vi "teleop.vi"() -> ()   [LabVIEW 2010]
uses:
  <vilib>/NXT/Dual Mode Library/Display/drawNumber.vi
  <vilib>/NXT/Dual Mode Library/Waits/Wait_Num.vi
  Remote Interface/Remote Interface.lvlib
panel:
  in  "Total Loops (lagometer)":i32
  out "Enabled?":enum16{"Disabled", "Enabled"}(ring)
types:
  T1 = typedef "LVHSConnector.ctl" = cluster{"Hardware":string, "Flattened String":string}
  T2 = cluster{"4134 Button ID":enum16{"1-1", "1-2", "1-3", "1-4", "1-5", "1-6", "1-7", "1-8", "1-9", "1-10", "1-11", "1-12", "2-1", "2-2", "2-3", "2-4", "2-5", "2-6", "2-7", "2-8", "2-9", "2-10", "2-11", "2-12", "NXT-L", "NXT-R", "NXT-E", "1-U", "1-UR", "1-R", "1-DR", "1-D", "1-DL", "1-L", "1-UL", "2-U", "2-UR", "2-R", "2-DR", "2-D", "2-DL", "2-L", "2-UL"}, "4134 Event Type":enum16{"Pressed", "Released", "Toggled", "Untoggled"}}[]
  T3 = enum16{"Pressed", "Released", "Toggled", "Untoggled"}
  T4 = enum16{"None", "Left Button", "Right Button", "Enter Button"}
  T5 = enum16{"None", "Button 1", "Button 2", "Button 3", "Button 4", "Button 5", "Button 6", "Button 7", "Button 8", "Button 9", "Button 10", "Button 11", "Button 12", "POV Up", "POV Up Right", "POV Right", "POV Down Right", "POV Down", "POV Down Left", "POV Left", "POV Up Left"}
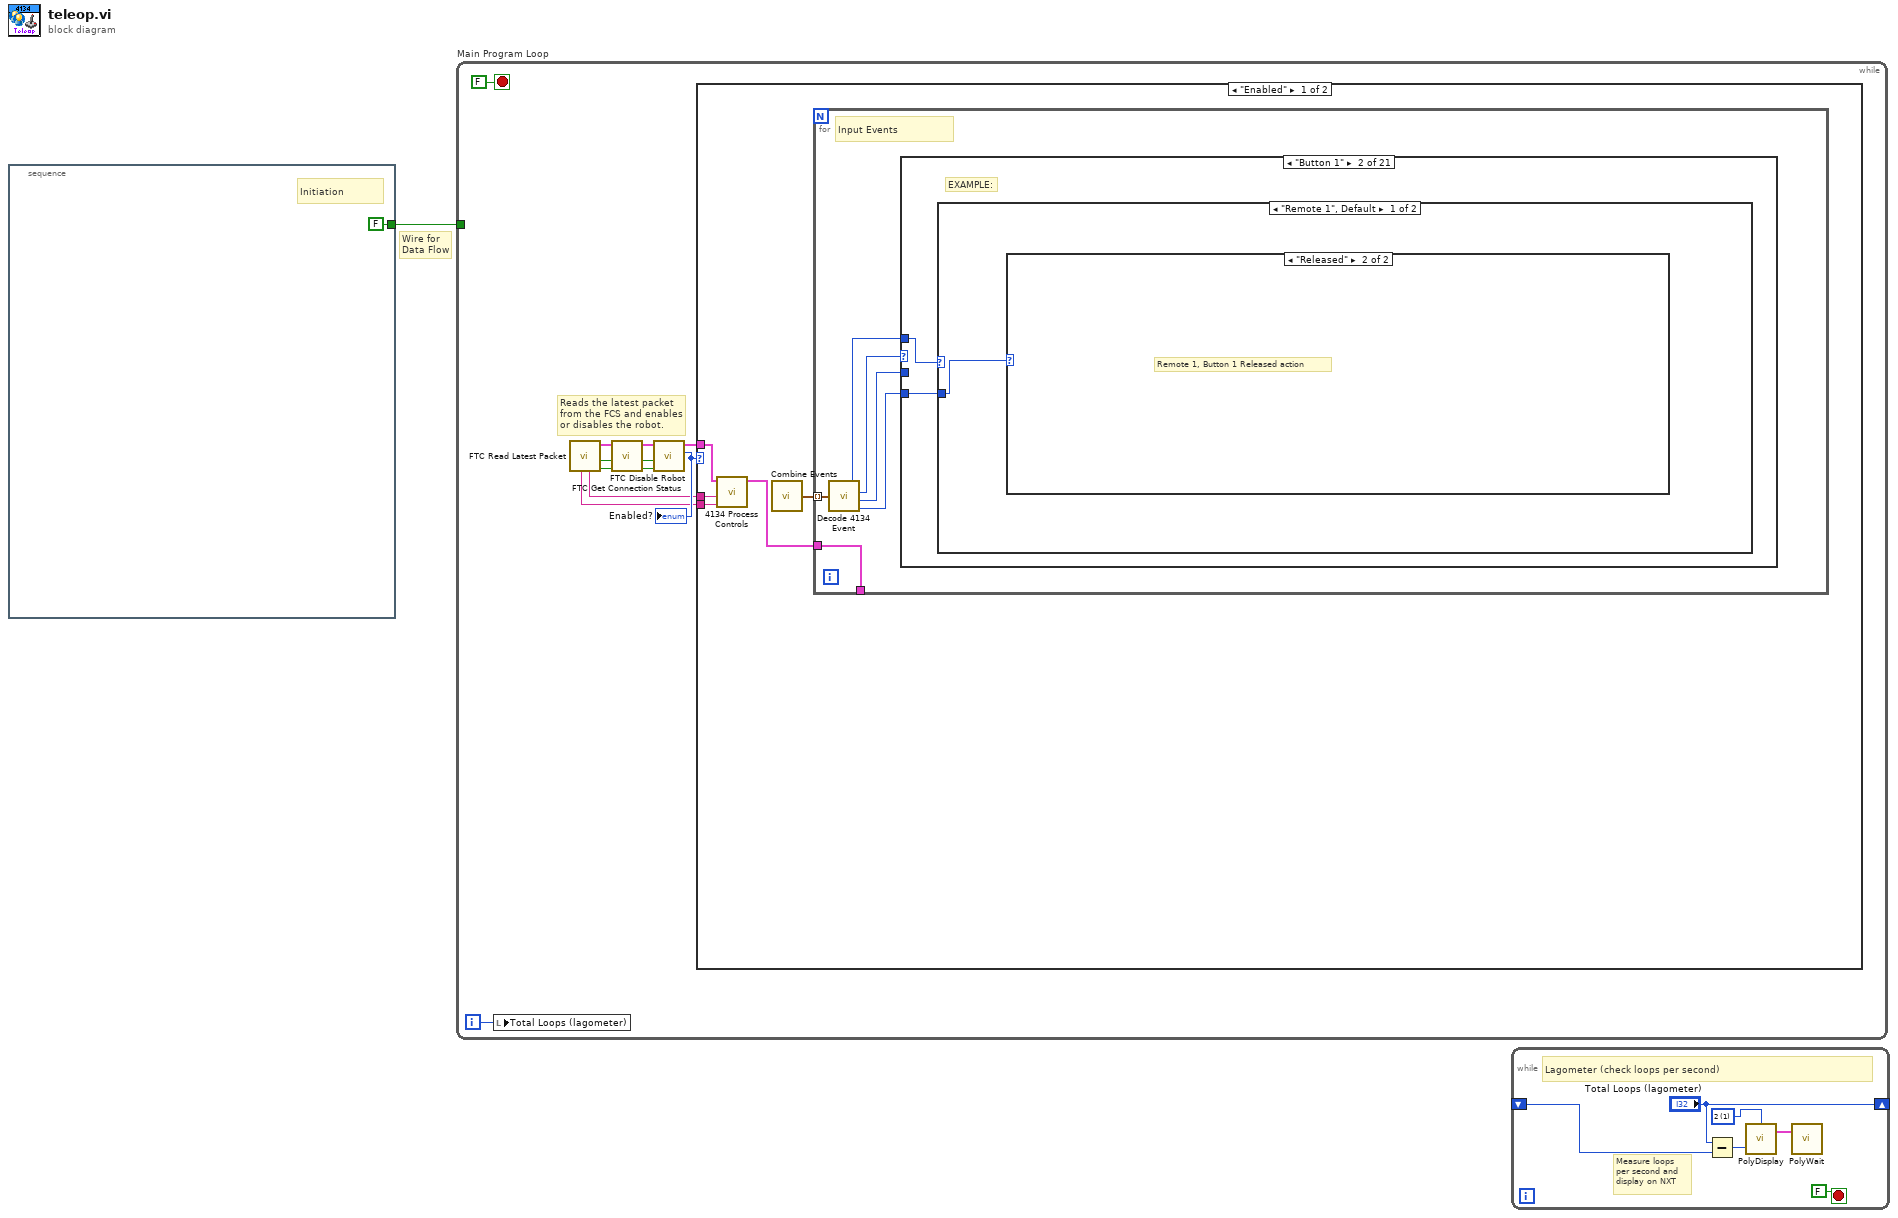
[diagram p0: block diagram]
diagram:
  # "Wire for\nData Flow"
  n1 = stacked-sequence {
    tunnel: [FALSE] -> w1
    frame #0 {
      # "Initiation"
    }
  }
  n2 = while "Main Program Loop" {
    tunnel: w1 -> [_]
    i -> [w3]
    stop <- FALSE stop-if-true
    # "Reads the latest packet\nfrom the FCS and enables\nor disables the robot."
    n3 = local write "Total Loops (lagometer)"(w3) -> ()
    n4 = call <vilib>:"FTC Read Latest Packet.vi"() -> ("Packet Received?"=w13:bool, "Stopped?"=w10:bool, "NXT"=w12:T1, "Controller 1"=w5:string, "Controller 2"=w4:string)  [unwired: 6 in, 1 out]
    n5 = call <vilib>:"FTC Get Connection Status.vi"("Packet Received?"=w13, "Stopped?"=w10, "NXT"=w12) -> ("Online?"=w7:bool, "Stopped?"=w8:bool, "NXT"=w9:T1)  [unwired: 5 in]
    n6 = call <vilib>:"FTC Disable Robot.vi"("Online?"=w7, "Stopped?"=w8, "NXT"=w9) -> ("Enabled?"=w11:enum16{"Disabled", "Enabled"}, "NXT"=w6:T1)  [unwired: 3 in]
    "Enabled?" <- w11
    n7 = case "disableCase" shown="\"Enabled\"" w11 {
      tunnel: w5 -> [w19 _]
      tunnel: w4 -> [w18 _]
      tunnel: w6 -> [w17 w34]
      frame "Enabled" {
        n8 = call "4134 Process Controls.vi"("Remote 2 Packet"=w18, "Remote 1 Packet"=w19, "NXT"=w17) -> ("NXT"=w15:T1)  [unwired: 6 in, 2 out]
        n9 = call "Combine Events.vi"() -> ("4134 Events"=w16:T2)  [unwired: 2 in]
        n10 = for {
          tunnel: w16 -> [w25] mode=indexing
          tunnel: w15 -> [w20]
          tunnel: [w20] -> _
          # "Input Events"
          n11 = call "Decode 4134 Event.vi"("4134 Event"=w25) -> ("4134 Event Type"=w22:T3, "NXT Button"=w23:T4, "FTC Button"=w24:T5, "Source"=w21:enum16{"NXT", "Remote 1", "Remote 2"})
          n12 = case shown="\"Button 1\"" w24 {
            tunnel: w23 -> [w27 _ _ _ _ _ _ _ _ _ _ _ _ _ _ _ _ _ _ _ _]
            tunnel: w22 -> [w26 w31 _ _ _ _ _ _ _ _ _ _ _ _ _ _ _ _ _ _ _]
            tunnel: w21 -> [w28 w32 _ _ _ _ _ _ _ _ _ _ _ _ _ _ _ _ _ _ _]
            frame "None", Default {
              n13 = case shown="\"NXT\"" w28 {
                tunnel: w27 -> [w30 _]
                tunnel: w26 -> [w29 _]
                frame "NXT" {
                  # "An NXT Button was pressed:"
                  n14 = case shown="\"None\", Default" w30 {
                    tunnel: w29 -> [_ _ _ _]
                    frame "None", Default {
                    }
                    frame "Left Button" {
                    }
                    frame "Right Button" {
                    }
                    frame "Enter Button" {
                    }
                  }
                }
                frame Default {
                  # "Invalid case, do nothing"
                }
              }
            }
            frame "Button 1" {
              # "EXAMPLE:"
              n15 = case shown="\"Remote 1\", Default" w32 {
                tunnel: w31 -> [w33 _]
                frame "Remote 1", Default {
                  n16 = case shown="\"Released\"" w33 {
                    frame "Pressed", Default {
                      # "Remote 1, Button 1 Pressed action"
                    }
                    frame "Released" {
                      # "Remote 1, Button 1 Released action"
                    }
                  }
                }
                frame "Remote 2" {
                }
              }
            }
            frame "Button 2" {
            }
            frame "Button 3" {
            }
            frame "Button 4" {
            }
            frame "Button 5" {
            }
            frame "Button 6" {
            }
            frame "Button 7" {
            }
            frame "Button 8" {
            }
            frame "Button 9" {
            }
            frame "Button 10" {
            }
            frame "Button 11" {
            }
            frame "Button 12" {
            }
            frame "POV Up" {
            }
            frame "POV Up Right" {
            }
            frame "POV Right" {
            }
            frame "POV Down Right" {
            }
            frame "POV Down" {
            }
            frame "POV Down Left" {
            }
            frame "POV Left" {
            }
            frame "POV Up Left" {
            }
          }
        }
      }
      frame "Disabled" {
        n17 = call <vilib>:"FTC Display Connection Status.vi"("NXT"=w34) -> ()  [unwired: 10 in, 1 out]
      }
    }
  }
  n18 = while {
    shift-right: ["Total Loops (lagometer)"] -> _
    shift-left: _ -> [w38]
    stop <- FALSE stop-if-true
    w39 = i16 1 items=["1", "2", "3", "4", "5", "6", "7", "8"] ("Line")
    # "Lagometer (check loops per second)"
    # "Measure loops\nper second and\ndisplay on NXT"
    n19 = Subtract(x="Total Loops (lagometer)", y=w38) -> (x-y=w37:i32)
    n20 = call-poly <vilib>:"PolyDisplay.vi"("number"=w37, "Line"=w39) -> ("NXT"=w35:T1)  [unwired: 2 in]
    n21 = call-poly <vilib>:"PolyWait.vi"("NXT"=w35) -> ()  [unwired: 3 in, 1 out]
  }
